vi "CSMLS - Define Loop State(s).vi"(0 "Loop States":string="Start\nLoop -><loop>\nStop\nFinish", 5 "States Queue":string, 9 "Add to Front? (F)":bool) -> (6 "Remaining States":string)   [LabVIEW 2017, in "CSM Loop Support.lvlib"]
doc: "Defines a loop operation, identifying the repeating loop state via the tag `-><loop>`. This loop also appends the `-><end>` tag at the end to mark the loop's conclusion.\n\nFor example, the following loop can be defined:\n\n DAQ: Initialize\n DAQ: Start\n DAQ: Continue Check -><loop> // Call the CSMLS - Append Continuous State VI in this loop to repeat acquisition and wait for a period as the loop interval.\n DAQ: Stop\n DAQ: Close -><end> // -><end> is automatically added.\n\nDuring the loop process, synchronous messages will interrupt the loop and execute immediately due to their high priority. Asynchronous messages have lower priority; after being dequeued, they are added after the `-><end>` tag. At this point, the CSMLS - Append Continuous State VI within `DAQ: Continue Check` will move the states after the `-><end>` tag to the front of the queue, thus allowing asynchronous messages to be responded to during the loop.\n\nThe loop can be ended by removing `-><loop>`. You can use the following VIs to remove the loop tag:\n- CSMLS - Remove Loop Tag and previous State(s) to Break VI: Removes the line containing the `-><loop>` tag and all preceding states, used to break out of the loop.\n- CSMLS - Remove Loop Tag to Break VI: Removes the line containing the `-><loop>` tag, used to break out of the loop.\n\n<b>Reference Example</b>: `Addons - Loop Support\\CSMLS - Continuous Loop in CSM Example.vi`.\n\n\n> [!NOTE] <b>Reason for CSM LOOP Support Design</b>\n>\n> A loop is the basic unit of operation for a state machine, executing continuously while the state machine is running. Users can define loop conditions via logic or use the CSM-recommended Loop Support Addon to define loops.\n>\n> Typically loop schemes may have the following issues:\n> - Implementing a loop within a Case branch can cause the state machine to get stuck in that state, unable to switch normally or respond to external messages.\n> - Inserting the next loop state in the last state of a state loop can also result in poor response to external messages and is unintuitive.\n>\n> The advantage of the way Loop Support defines loops is that it can still respond to other events while the loop is running, without blocking the operation of the state machine. CSM Loop-Support VIs are used to define, append, and terminate loops, using special tags to identify the corresponding loop states and the end state. Therefore, this addon is primarily intended to provide a standard loop implementation method to solve the above problems.\n\n\n> [!WARNING] <b>CSM LOOP Support Applicability</b>\n>\n> The CSM collaborator (worker) and chain modes are special module patterns composed of multiple running nodes. Messages sent in these modes cannot reliably target a specific node to execute. When a node operates in collaborator (worker) or chain modes, it cannot be clearly instructed by messages to stop a loop. Therefore, it is not recommended to use the CSM Loop Support addon in collaborator (worker) and chain modes.\n\n\n> [!WARNING]\n> <b>Add to Front? (F)</b> is usually FALSE because once a loop state starts, it does not end immediately. Before insertion into the state queue, it is considered a sub-state of the current state. If the current state was called via a synchronous message, it would not return immediately. For example, if a set of continuous acquisition states is defined in `API: Start DAQ` and this message is sent synchronously from outside, the logic should be to start the loop and then return immediately. Only set <b>Add to Front? (F)</b> to TRUE if the logic is to wait for the loop to end before returning.\n\n> [!WARNING]\n> Be careful not to connect <b>State Queue</b> and <b>Loop States</b> in reverse. If reversed, it may cause synchronous messages sent externally to fail to return, and external messages can no longer be processed.\n\n-- <b>Controls</b> --\n- <b>States Queue</b>: Connect the entire state queue to this input.\n- <b>Loop States</b>: Loop states.\n- <b>Add to Front? (F)</b>: Whether to add to the front of all states. The default is FALSE.\n\n-- <b>Indicators</b> --\n- <b>Remaining States</b>: The processed message queue."
uses:
  CSM Loop Support.lvlib
  Communicable State Machine.lvlib
  _Shared/CSM Shared.lvlib
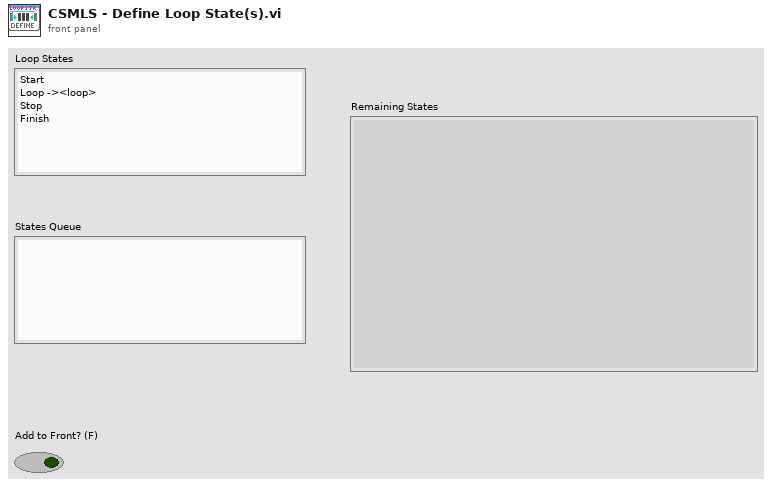
[diagram p1: front panel]
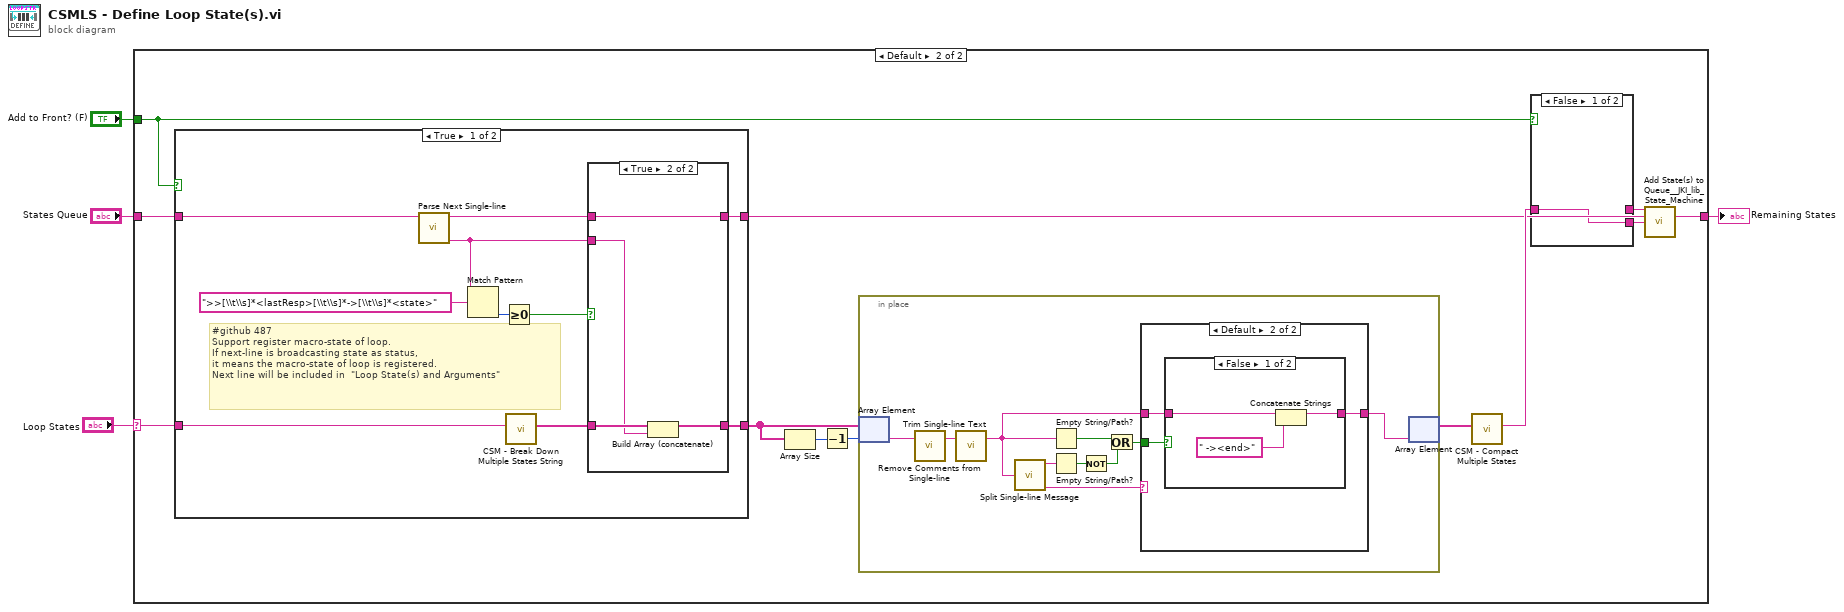
[diagram p0: block diagram]
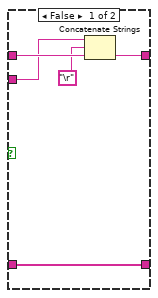
[diagram p3: hidden frame]
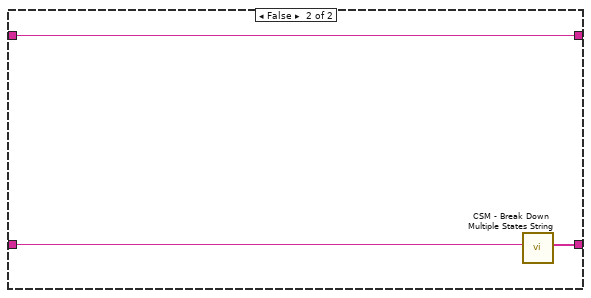
[diagram p4: hidden frame]
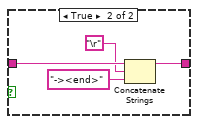
[diagram p7: hidden frame]
diagram:
  n1 = case shown="Default" "Loop States" {
    selector: "Loop States" -> [_ w16]
    tunnel: [w5 w17] -> w4
    tunnel: "States Queue" -> [w5 w15]
    tunnel: "Add to Front? (F)" -> [_ w6]
    frame "" {
    }
    frame Default {
      n2 = case shown="True" w6 {
        tunnel: w16 -> [w27 w39]
        tunnel: w15 -> [w26 w37]
        tunnel: [w22 w38] -> w8
        tunnel: [w19 w37] -> w7
        frame True {
          # "#github 487\nSupport register macro-state of loop.\nIf next-line is broadcasting state as status,\nit means the macro-state of loop is registered.\nNext line will be included in  \"Loop State(s) and Arguments\""
          n3 = call "Parse Next Single-line.vi"("States Queue"=w26) -> ("Next Single-line State"=w21:string, "Remaining States Queue"=w18:string)  [unwired: 9 in]
          n4 = Match Pattern(string=w21, regular expression=">>[\\t\\s]*<lastResp>[\\t\\s]*->[\\t\\s]*<state>") -> (offset past match=w23:i32)  [unwired: 1 in, 3 out]
          n5 = Greater Or Equal To 0?(x=w23) -> (x >= 0?=w20:bool)
          n6 = call "CSM - Break Down Multiple States String.vi"("States"=w27) -> ("Multiple States"=w25:string[])  [unwired: 10 in]
          n7 = case shown="True" w20 {
            tunnel: w25 -> [w32 w36]
            tunnel: [w32 w35] -> w22
            tunnel: w21 -> [w29 w34]
            tunnel: [w30 w33] -> w19
            tunnel: w18 -> [w31 w33]
            frame False {
              n8 = Concatenate Strings(w29, "\r", w31) -> (w30:string)
            }
            frame True {
              n9 = Build Array (concatenate)(w36, w34) -> (w35:string[])
            }
          }
        }
        frame False {
          n10 = call "CSM - Break Down Multiple States String.vi"("States"=w39) -> ("Multiple States"=w38:string[])  [unwired: 10 in]
        }
      }
      n11 = Array Size(array=w8) -> (size(s)=w11:i32)
      n12 = Decrement(x=w11) -> (x-1=w10:i32)
      n13 = in-place {
        n14 = in-place-array #1(w8, w10) -> (w43:string)
        n15 = call "Remove Comments from Single-line.vi"("single-line text"=w43) -> ("single-line text without comments"=w46:string)  [unwired: 2 in]
        n16 = call "Trim Single-line Text.vi"("single-line text"=w46) -> ("trimed text"=w45:string)  [unwired: 2 in]
        n17 = call "Split Single-line Message.vi"("single-line text"=w45) -> ("operator"=w51:string, "source/target"=w44:string)  [unwired: 6 in, 2 out]
        n18 = Empty String/Path?(string/path=w45) -> (empty?=w49:bool)
        n19 = Empty String/Path?(string/path=w51) -> (empty?=w50:bool)
        n20 = Not(x=w50) -> (.not. x?=w48:bool)
        n21 = Or(x=w49, y=w48) -> (x .or. y?=w47:bool)
        n22 = case shown="Default" w44 {
          tunnel: w47 -> [_ w55]
          tunnel: [w52 w54] -> w42
          tunnel: w45 -> [w52 w53]
          frame "<end>" {
          }
          frame Default {
            n23 = case shown="False" w55 {
              tunnel: w53 -> [w57 w62]
              tunnel: [w56 w59] -> w54
              frame False {
                n24 = Concatenate Strings(w57, " -><end>" ("string")) -> (w56:string)
              }
              frame True {
                n25 = Concatenate Strings(w62, "\r", "-><end>" ("string")) -> (w59:string)
              }
            }
          }
        }
        n26 = in-place-array #1(w42) -> (w9:string[])  [unwired: 1 out]
      }
      n27 = call "CSM - Compact Multiple States.vi"("Multiple States"=w9) -> ("States"=w14:string)  [unwired: 9 in]
      n28 = case shown="False" w6 {
        tunnel: w14 -> [w40 w41]
        tunnel: [_ w41] -> w13
        tunnel: [w40 _] -> w12
        frame False {
        }
        frame True {
        }
      }
      n29 = call <vilib>:"Add State(s) to Queue__JKI_lib_State_Machine.vi"("State(s) in Front (\"\")"=w13, "State(s) in (\"\")"=w7, "State(s) at Back (\"\")"=w12) -> ("States Out"=w17:string)  [unwired: 12 in]
    }
  }
  "Remaining States" <- w4
